vi "HO -Group on.vi"(1 "Group #":i8=1 min=1 max=6 step=1, 3 "error in":errorcluster, 4 "Action":bool, 5 "Address / Port":i16=1 min=1 max=31 step=1) -> (0 "error out":errorcluster, 2 "Query group power\nStatus - read":dbl format="%.2f")   [LabVIEW 2014]
panel:
  # "Read"
  # "Write"
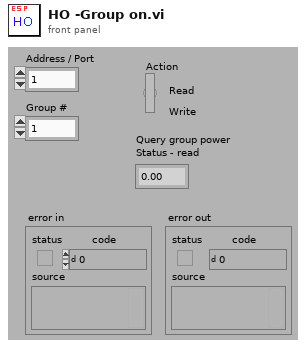
[diagram p1: front panel]
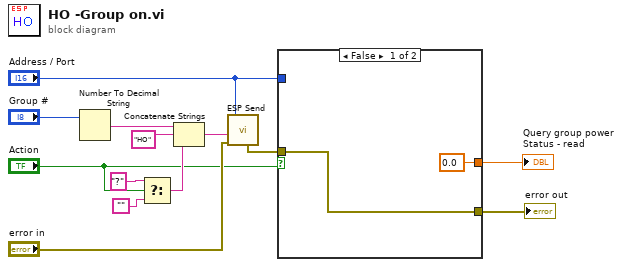
[diagram p0: block diagram]
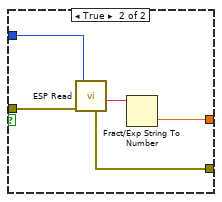
[diagram p2: hidden frame]
diagram:
  n1 = Number To Decimal String(number="Group #") -> (decimal integer string=w12:string)  [unwired: 1 in]
  n2 = Select(t="?", s="Action", f="") -> (s? t:f=w9:string)
  n3 = Concatenate Strings(w12, "HO" ("Substring"), w9) -> (w10:string)
  n4 = call "ESP Send.vi"("Address / Port"="Address / Port", "Command String"=w10, "error in"="error in") -> ("error out"=w4:errorcluster)  [unwired: 5 in]
  n5 = case shown="False" "Action" {
    tunnel: "Address / Port" -> [_ w20]
    tunnel: w4 -> [w15 w19]
    tunnel: [w15 w18] -> w3
    tunnel: [0.0 w16] -> w2
    frame False {
    }
    frame True {
      n6 = call "ESP Read.vi"("Address / Port"=w20, "error in"=w19) -> ("error out"=w18:errorcluster, "Response String"=w17:string)  [unwired: 5 in]
      n7 = Fract/Exp String To Number(string=w17) -> (number=w16:dbl)  [unwired: 3 in, 1 out]
    }
  }
  "error out" <- w3
  "Query group power\nStatus - read" <- w2
